vi "InbetweenDist2point.vi"(6 "Posit Array":T1[](array[typedef]), 7 "Inbetween diff":dbl=5.0, 10 "Index":i32, 11 "All Lines":T2) -> (0 "Bad   In angle?":bool, 1 "Lower index":i32, 2 "In range?":bool)   [LabVIEW 2014]
uses:
  Libraries/Map Data Folder/All-Lines.ctl
  Libraries/Map Data Folder/LineCluster.ctl
  Libraries/Map Data Folder/LineConnection.ctl
  Libraries/Contact Data/Position.ctl
  Libraries/Map Data Folder/Map Data.lvlib
  Libraries/Contact Data/Contact Data.lvlib
panel:
  in  "Less than":dbl=100.0
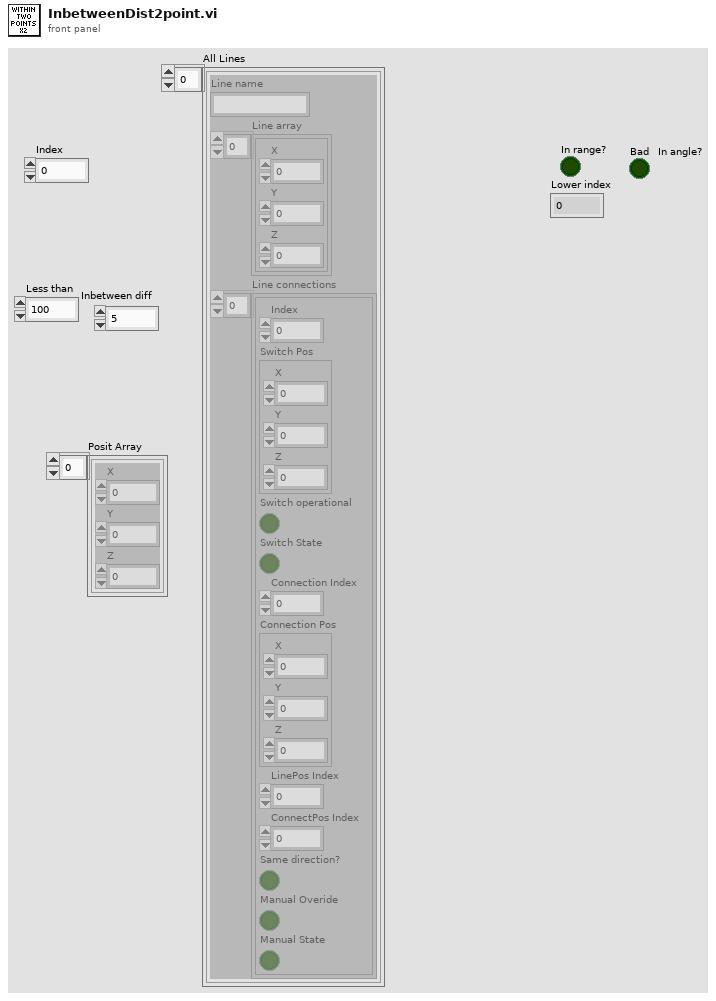
[diagram p1: front panel]
types:
  T1 = typedef "Contact Data.lvlib/Position.ctl" = cluster{"X":dbl, "Y":dbl, "Z":dbl}
  T2 = typedef "Map Data.lvlib/All-Lines.ctl" = T3[]
  T3 = typedef "Map Data.lvlib/LineCluster.ctl" = cluster{"Line name":string, "Line array":cluster{"X":dbl, "Y":dbl, "Z":dbl}[], "Line connections":T4[]}
  T4 = typedef "Map Data.lvlib/LineConnection.ctl" = cluster{"Index":i32, "Switch Pos":cluster{"X":dbl, "Y":dbl, "Z":dbl}, "Switch operational":bool, "Switch State":bool, "Connection Index":i32, "Connection Pos":cluster{"X":dbl, "Y":dbl, "Z":dbl}, "LinePos Index":i32, "ConnectPos Index":i32, "Same direction?":bool, "Manual Overide":bool, "Manual State":bool}
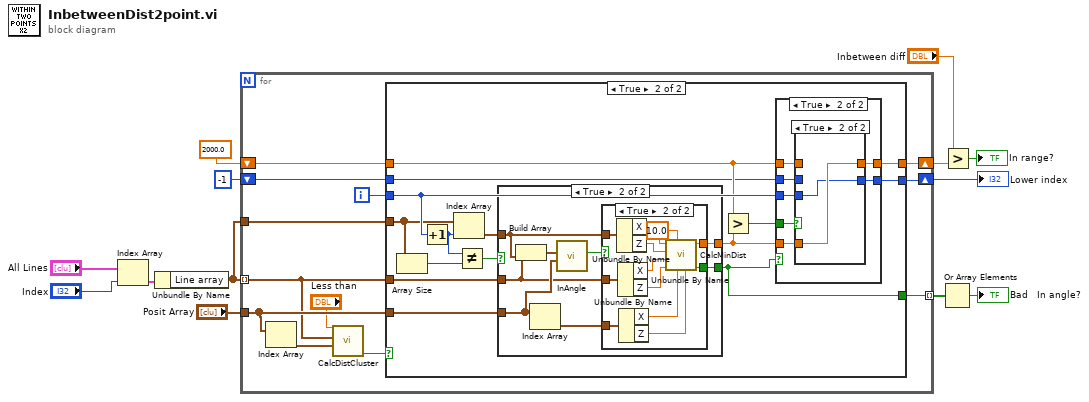
[diagram p0: block diagram]
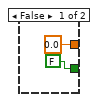
[diagram p3: hidden frame]
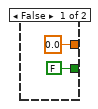
[diagram p4: hidden frame]
diagram:
  n1 = Index Array(array="All Lines", index="Index") -> (element=w13:T3)
  n2 = Unbundle By Name(w13) -> ("Line array"=w10:cluster{"X":dbl, "Y":dbl, "Z":dbl}[])
  n3 = for {
    tunnel: w10 -> [w16] mode=indexing
    tunnel: w10 -> [w20]
    shift-right: [w24] -> w8
    shift-left: 2000.0 ("Result") -> [w23]
    shift-right: [w22] -> w4
    shift-left: -1 -> [w21]
    tunnel: [w19] -> w3 mode=indexing
    tunnel: "Posit Array" -> [w18]
    i -> [w25]
    n4 = Index Array(array=w18) -> (element=w17:T1)  [unwired: 1 in]
    n5 = call "CalcDistCluster.vi"("Less than"="Less than", "element 2"=w17, "element"=w16) -> ("Less than?"=w14:bool)  [unwired: 7 in, 1 out]
    n6 = case shown="True" w14 {
      selector: w14 -> [w26 _]
      tunnel: w25 -> [_ w43]
      tunnel: [w27 w41] -> w24
      tunnel: w23 -> [w27 w40]
      tunnel: [w28 w38] -> w22
      tunnel: w21 -> [w28 w37]
      tunnel: w20 -> [_ w35]
      tunnel: [w26 w32] -> w19
      tunnel: w18 -> [_ w30]
      tunnel: w16 -> [_ w29]
      frame False {
      }
      frame True {
        n7 = Array Size(array=w35) -> (size(s)=w31:i32)
        n8 = Increment(x=w43) -> (x+1=w33:i32)
        n9 = Index Array(array=w35, index=w33) -> (element=w36:cluster{"X":dbl, "Y":dbl, "Z":dbl})
        n10 = Not Equal?(x=w33, y=w31) -> (x != y?=w34:bool)
        n11 = case shown="True" w34 {
          tunnel: w29 -> [_ w47]
          tunnel: [0.0 ("Result") w53] -> w42
          tunnel: w36 -> [_ w46]
          tunnel: [FALSE ("Inbetween?") w52] -> w32
          tunnel: w30 -> [_ w49]
          frame False {
          }
          frame True {
            n12 = Build Array(w47, w46) -> (w51:cluster{"X":dbl, "Y":dbl, "Z":dbl}[])
            n13 = Index Array(array=w49) -> (element=w48:T1)  [unwired: 1 in]
            n14 = call "InAngle.vi"("2nd Array (Start)"=w49, "Base Array (End)"=w51) -> ("In Angle?"=w50:bool)  [unwired: 9 in]
            n15 = case shown="True" w50 {
              tunnel: [0.0 ("Result") w63] -> w53
              tunnel: [FALSE ("In Angle?") w62] -> w52
              tunnel: w46 -> [_ w61]
              tunnel: w47 -> [_ w60]
              tunnel: w48 -> [_ w59]
              frame False {
              }
              frame True {
                n16 = Unbundle By Name(w61) -> ("X"=w65:dbl, "Z"=w64:dbl)
                n17 = Unbundle By Name(w60) -> ("X"=w67:dbl, "Z"=w66:dbl)
                n18 = Unbundle By Name(w59) -> ("X"=w58:dbl, "Z"=w57:dbl)
                n19 = call "CalcMinDist.vi"("PointY"=w57, "PointX"=w58, "Angle"=10.0, "Line2Y"=w66, "Line2X"=w67, "Line1Y"=w64, "Line1X"=w65) -> ("In Angle?"=w62:bool, "Result"=w63:dbl)  [unwired: 3 in]
              }
            }
          }
        }
        n20 = Greater?(x=w40, y=w42) -> (0:w39:bool)
        n21 = case shown="True" w32 {
          tunnel: w42 -> [_ w75]
          tunnel: w43 -> [_ w71]
          tunnel: w40 -> [w69 w73]
          tunnel: [w69 w74] -> w41
          tunnel: w39 -> [_ w76]
          tunnel: [w68 w72] -> w38
          tunnel: w37 -> [w68 w70]
          frame False {
          }
          frame True {
            n22 = case shown="True" w76 {
              tunnel: w75 -> [_ w80]
              tunnel: [w78 w80] -> w74
              tunnel: w73 -> [w78 _]
              tunnel: [w77 w79] -> w72
              tunnel: w71 -> [_ w79]
              tunnel: w70 -> [w77 _]
              frame False {
              }
              frame True {
              }
            }
          }
        }
      }
    }
  }
  "Lower index" <- w4
  n23 = Or Array Elements(Boolean array=w3) -> (logical OR=→"Bad   In angle?":bool)
  n24 = Greater?(x="Inbetween diff", y=w8) -> (0:→"In range?":bool)
